vi "letras.vi"() -> ()   [LabVIEW 2016]
panel:
  out "substring":string
  out "Array":bool[](array[boolean])
  in  "String":string
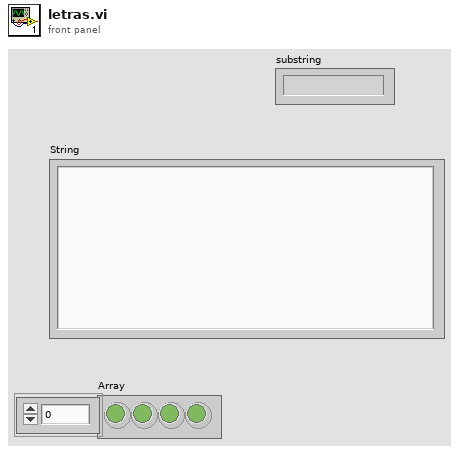
[diagram p1: front panel]
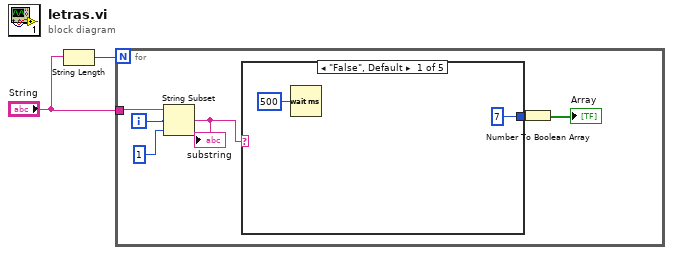
[diagram p0: block diagram]
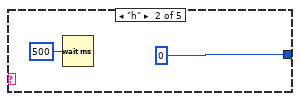
[diagram p2: hidden frame]
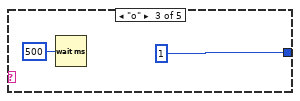
[diagram p3: hidden frame]
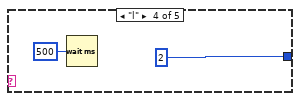
[diagram p4: hidden frame]
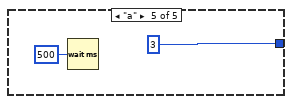
[diagram p5: hidden frame]
diagram:
  n1 = String Length(string="String") -> (length=w1:i32)
  n2 = for {
    N: w1 -> [_]
    tunnel: "String" -> [w8]
    i -> [w6]
    n3 = String Subset(string=w8, offset (0)=w6, length (rest)=1 ("length (rest)")) -> (substring=w5:string)
    "substring" <- w5
    n4 = case shown="\"False\", Default" w5 {
      tunnel: [7 0 1 2 3] -> w4
      frame "False", Default {
        n5 = Wait (ms)(milliseconds to wait=u32 500) -> ()  [unwired: 1 out]
      }
      frame "h" {
        n6 = Wait (ms)(milliseconds to wait=u32 500) -> ()  [unwired: 1 out]
      }
      frame "o" {
        n7 = Wait (ms)(milliseconds to wait=u32 500) -> ()  [unwired: 1 out]
      }
      frame "l" {
        n8 = Wait (ms)(milliseconds to wait=u32 500) -> ()  [unwired: 1 out]
      }
      frame "a" {
        n9 = Wait (ms)(milliseconds to wait=u32 500) -> ()  [unwired: 1 out]
      }
    }
    n10 = Number To Boolean Array(number=w4) -> (Boolean array=→"Array":bool[])
  }
